vi "CPP_MultiProbe.vi"(4 "Pressure (mBar)":dbl=1000.0, 5 "Temperature (C)":dbl=20.0, 6 "Old5HoleProbe?":bool, 7 "Calibration Folder Path":path=path "G:/5HoleProbe", 9 "ZeroedPressures (mmH2O)":dbl[][](array[numeric])=array820x5[4100 elements]) -> (0 "Time (ms)":u32, 1 "TotalPoints":i32, 2 "ReductionCode":i32[](array[numeric]), 3 "RawVmagUVWCone":dbl[][](array[numeric]))   [LabVIEW 2015]
uses:
  VWflipperScalar.vi
panel:
  out "Progress":dbl(slide)=819.0 max=820.0 scale=-1.0..820.0
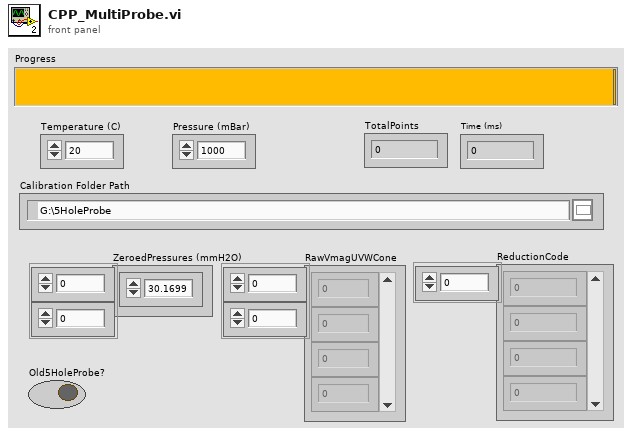
[diagram p1: front panel]
types:
  T1 = cluster{"[0]":dbl, "[1]":dbl, "[2]":dbl, "[3]":dbl, "[4]":dbl}
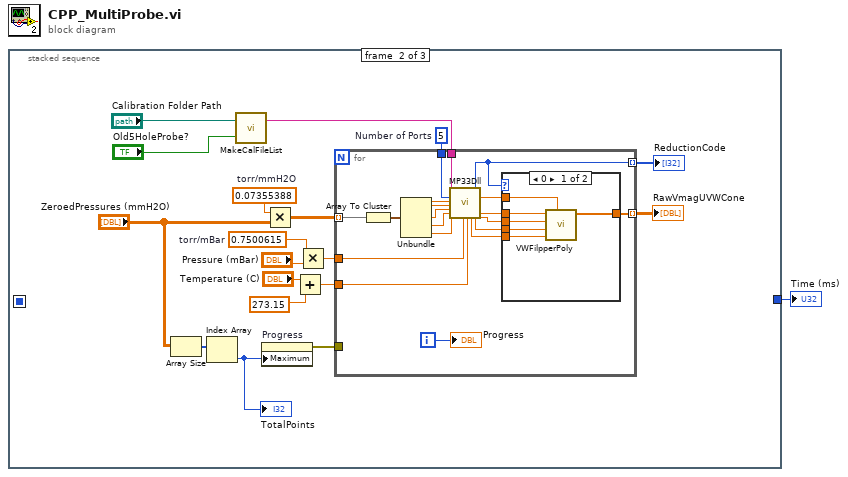
[diagram p0: block diagram]
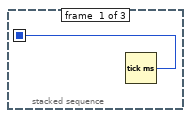
[diagram p2: hidden frame]
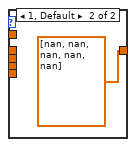
[diagram p3: hidden frame]
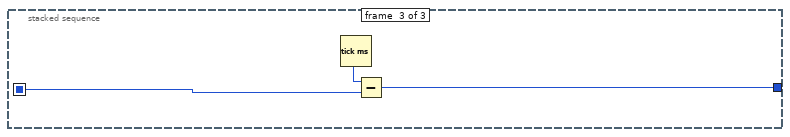
[diagram p4: hidden frame]
diagram:
  n1 = stacked-sequence {
    seq-local: [w2 _ _] -> [_ _ w47]
    tunnel: [_ _ w49] -> w1
    frame #0 {
      n2 = Tick Count (ms)() -> (millisecond timer value=w2:u32)
    }
    frame #1 {
      w18 = 0.7500615  # torr/mBar
      w11 = 0.07355388  # torr/mmH2O
      w3 = 5  # Number of Ports
      n3 = Array Size(array="ZeroedPressures (mmH2O)") -> (size(s)=w5:i32[])
      n4 = Index Array(array=w5) -> (element=w7:i32)  [unwired: 1 in]
      "TotalPoints" <- w7
      n5 = call "MakeCalFileList.vi"("Old5HoleProbe?"="Old5HoleProbe?", "Calibration Folder Path"="Calibration Folder Path") -> ("MultiProbeCals"=w10:string)  [unwired: 1 out]
      n6 = property on="Progress" class="Slide (strict)"("Maximum"=w7) -> (error out=w4:errorcluster)  [unwired: 2 in, 1 out]
      n7 = Multiply(x=w11, y="ZeroedPressures (mmH2O)") -> (x*y=w13:dbl[][])
      n8 = Add(x="Temperature (C)", y=273.15 ("x")) -> (x+y=w16:dbl)
      n9 = Multiply(x=w18, y="Pressure (mBar)") -> (x*y=w19:dbl)
      n10 = for {
        tunnel: [w28] -> w6 mode=indexing
        tunnel: w3 -> [w33]
        tunnel: w19 -> [w32]
        tunnel: w4 -> [_]
        tunnel: w10 -> [w24]
        tunnel: w13 -> [w23] mode=indexing
        tunnel: [w21] -> w14 mode=indexing
        tunnel: w16 -> [w22]
        i -> [w27]
        n11 = Array To Cluster(array=w23) -> (cluster=w39:T1)
        n12 = Unbundle(w39) -> ("[0]"=w38:dbl, "[1]"=w37:dbl, "[2]"=w36:dbl, "[3]"=w35:dbl, "[4]"=w34:dbl)
        n13 = call "MP33Dll.vi"("MultiProbeCals"=w24, "Number of Ports"=w33, "P1 Torr"=w38, "P2 Torr"=w37, "P3 Torr"=w36, "P4 Torr"=w35, "P5 Torr"=w34, "Pref Torr"=w32, "TTot Kelvin"=w22) -> ("w m/s"=w29:dbl, "return type"=w21:i32, "v m/s"=w30:dbl, "Theta Degree"=w25:dbl, "VMagn m/s"=w31:dbl, "u  m/s"=w26:dbl)  [unwired: 8 in, 5 out]
        n14 = case shown="0" w21 {
          tunnel: w31 -> [w45 _]
          tunnel: w30 -> [w44 _]
          tunnel: w29 -> [w43 _]
          tunnel: [w42 dbl[] [nan, nan, nan, nan, nan] ("VmagUVWCone")] -> w28
          tunnel: w26 -> [w41 _]
          tunnel: w25 -> [w40 _]
          frame 0 {
            n15 = call-poly "VWFilpperPoly.vi"("Theta Degree"=w40, "Probe w m/s"=w43, "Probe v m/s"=w44, "Probe u  m/s"=w41, "VMagn m/s"=w45) -> ("VmagUVWCone"=w42:dbl[])  [unwired: 6 in]
          }
          frame 1, Default {
          }
        }
        "Progress" <- w27
      }
      "RawVmagUVWCone" <- w6
      "ReductionCode" <- w14
    }
    frame #2 {
      n16 = Tick Count (ms)() -> (millisecond timer value=w48:u32)
      n17 = Subtract(x=w48, y=w47) -> (x-y=w49:u32)
    }
  }
  "Time (ms)" <- w1
